vi "Slewing Test SAA.vi"(8 "error in (no error)":errorcluster, 10 "Model in":refnum<class "Model.lvclass">, 11 "Test Actuator State in":refnum<class "Test Actuator State.lvclass">) -> (0 "error out":errorcluster, 1 "Pass":bool, 2 "Model out":refnum<class "Model.lvclass">, 3 "Test Actuator State out":refnum<class "Test Actuator State.lvclass">)   [LabVIEW 2016, in "Test Actuator State.lvclass"]
uses:
  Test Actuator State.lvclass
  Model/Model/Model.lvclass
  <vilib>/Platform/TimedLoop/XDataNode/timing_clust.ctl
  <vilib>/Platform/TimedLoop/XDataNode/nitl_modes.ctl
  <vilib>/Platform/TimedLoop/XDataNode/wakeup.ctl
  Model/Model/Model.lvclass/Model.ctl
  Typedefs/ActuatorSetPoints.ctl
  <vilib>/Analysis/baseanly.llb/Mean (DBL).vi
  <vilib>/platform/TimedLoop/XDataNode/XDataNode.xnode
  Model/Waveforms/Waveform/Waveform.lvclass
  Typedefs/FAMT Typedefs.lvlib
  <vilib>/Analysis/NI_AALBase.lvlib
  <vilib>/Platform/TimedLoop/XDataNode/XDNodeRunTimeDep.lvlib
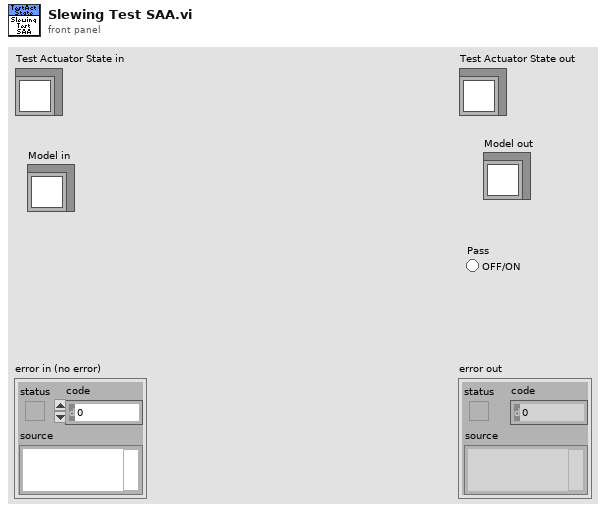
[diagram p1: front panel]
types:
  T1 = typedef "FAMT Typedefs.lvlib/SlewingTestSettings.ctl" = cluster{"Max Force Error (N)":dbl, "Max Moment (NM)":dbl, "Amplitude (N)":dbl, "Max Instance Force Error (N)":dbl, "Ramp Time (s)":dbl, "Hold Time (s)":dbl, "Settling Time (s)":dbl}
  T2 = typedef "XDNodeRunTimeDep.lvlib/timing_clust.ctl" = cluster{"Expected End [f-1]":u64, "Actual End [f-1]":u64, "Finished Late? [f-1]":bool, "Expected End [i-1]":u64, "Actual End [i-1]":u64, "Finished Late? [i-1]":bool, "Expected Start [i]":u64, "Actual Start [i]":u64, "Expected Start [f]":u64, "Actual Start [f]":u64, "Source Name":string, "Structure Name":string, "Period":i64, "Deadline":i64, "Offset":i64, "Start":i64, "Priority":i32, "Timeout":i32, "Mode":T3, "Wakeup Reason":T4, "Error":errorcluster, "Source Type":string, "Secondary Source Type":string, "Global End Time":u64, "Global Start Time":u64, "Frame Duration":u64, "Iteration Duration":u64, "Assigned CPU":i32, "I/O Scan Engine Mode":u32}
  T3 = typedef "XDNodeRunTimeDep.lvlib/nitl_modes.ctl" = enum32{"No Change", "Process missed periods, maintain original phase", "Discard missed periods, maintain original phase", "Process missed periods, ignore original phase", "Discard missed periods, ignore original phase"}
  T4 = typedef "XDNodeRunTimeDep.lvlib/wakeup.ctl" = enum32{"Normal", "Aborted", "Asynchronous wakeup", "Timing source error", "Timed loop error", "Timeout"}
  T5 = typedef "FAMT Typedefs.lvlib/ActuatorSetPoints.ctl" = cluster{"Axial Force":dbl, "Lateral Force":dbl, "FC1 Force":dbl, "FC2 Force":dbl}
  T6 = typedef "FAMT Typedefs.lvlib/ActuatorData.ctl" = cluster{"Timestamp":dbl, "Axial Force":dbl, "Lateral Force":dbl, "FC1 Force":dbl, "FC2 Force":dbl, "Lateral Push Pressure":dbl, "Lateral Pull Pressure":dbl, "Axial Push Pressure":dbl, "Axial Pull Pressure":dbl}
  T7 = typedef "FAMT Typedefs.lvlib/ToveyEngData.ctl" = cluster{"Timestamp":dbl, "Fx":dbl, "Fy":dbl, "Fz":dbl, "Mx":dbl, "My":dbl, "Mz":dbl}
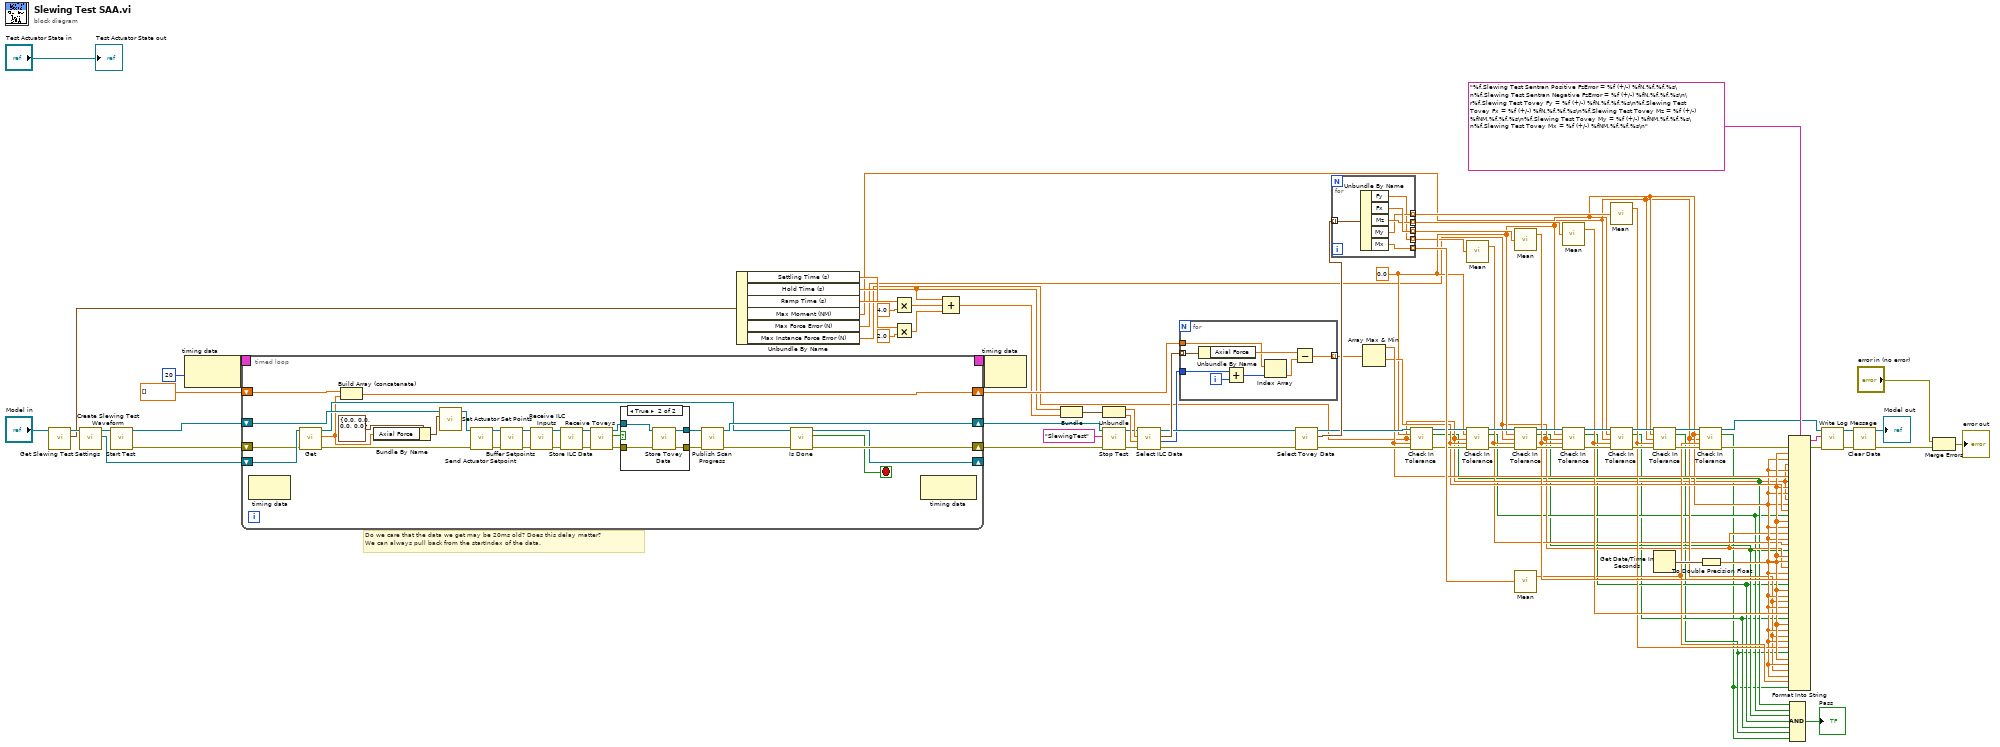
[diagram p0: block diagram]
diagram:
  w24 = 0.0
  # "Do we care that the data we get may be 20ms old? Does this delay matter?\nWe can always pull back from the startIndex of the data."
  n1 = call "Get Slewing Test Settings.vi"("Model in"="Model in") -> ("Slewing Test Settings"=w81:T1, "Model out"=w82:refnum<class "Model.lvclass">)  [unwired: 9 in]
  n2 = call "Create Slewing Test Waveform.vi"("Model in"=w82) -> ("Waveform"=w78:refnum<class "Waveform.lvclass">, "Model out"=w1:refnum<class "Model.lvclass">)  [unwired: 9 in]
  n3 = call "Start Test.vi"("Model in"=w1) -> ("error out"=w15:errorcluster, "Model out"=w16:refnum<class "Model.lvclass">)  [unwired: 9 in]
  n4 = node-c288(i64 20 ("Period")) -> (w73:T2)
  n5 = timed-loop {
    shift-right: [w113] -> w14
    shift-left: w16 -> [w105]
    shift-right: [w96] -> w13
    shift-left: w15 -> [w99]
    shift-right: [w94] -> _
    shift-left: w78 -> [w101]
    shift-right: [w91] -> w74
    shift-left: dbl[] [] -> [w93]
    timing: w73 -> [_]
    timing-out: [_] -> w72
    stop <- w95 stop-if-true
    n6 = node-c288() -> ()  [unwired: 1 in, 1 out]
    n7 = call-dynamic "Get.vi"("error in (no error)"=w99, "Waveform in"=w101) -> ("error out"=w98:errorcluster, "Value"=w92:dbl, "Waveform out"=w100:refnum<class "Waveform.lvclass">)  [unwired: 7 in]
    n8 = Build Array (concatenate)(w93, w92) -> (w91:dbl[])
    n9 = Bundle By Name(cluster=T5 {"Axial Force"=0.0, "Lateral Force"=0.0, "FC1 Force"=0.0, "FC2 Force"=0.0} ("Actuator Set Points"), "Axial Force"=w92) -> (w102:T5)
    n10 = call "Set Actuator Set Points.vi"("Actuator Set Points"=w102, "Model in"=w105) -> ("Model out"=w104:refnum<class "Model.lvclass">)  [unwired: 9 in]
    n11 = call "Send Actuator Setpoint.vi"("error in (no error)"=w98, "Model in"=w104) -> ("error out"=w88:errorcluster, "Model out"=w90:refnum<class "Model.lvclass">)  [unwired: 8 in]
    n12 = call "Buffer Setpoints.vi"("error in (no error)"=w88, "Model in"=w90) -> ("error out"=w87:errorcluster, "Model out"=w89:refnum<class "Model.lvclass">)  [unwired: 8 in]
    n13 = call "Receive ILC Inputs.vi"("error in (no error)"=w87, "Model in"=w89) -> ("error out"=w114:errorcluster, "Model out"=w115:refnum<class "Model.lvclass">)  [unwired: 8 in]
    n14 = call "Store ILC Data.vi"("error in (no error)"=w114, "Model in"=w115) -> ("error out"=w111:errorcluster, "Model out"=w112:refnum<class "Model.lvclass">)  [unwired: 8 in]
    n15 = call "Receive Toveys.vi"("error in (no error)"=w111, "Model in"=w112) -> ("error out"=w109:errorcluster, "Data Received"=w108:bool, "Model out"=w110:refnum<class "Model.lvclass">)  [unwired: 7 in]
    n16 = case shown="True" w108 {
      tunnel: w110 -> [w119 w123]
      tunnel: w109 -> [w118 w122]
      tunnel: [w118 w121] -> w106
      tunnel: [w119 w120] -> w107
      frame False {
      }
      frame True {
        n17 = call "Store Tovey Data.vi"("error in (no error)"=w122, "Model in"=w123) -> ("error out"=w121:errorcluster, "Model out"=w120:refnum<class "Model.lvclass">)  [unwired: 8 in]
      }
    }
    n18 = call "Publish Scan Progress.vi"("error in (no error)"=w106, "Model in"=w107) -> ("error out"=w97:errorcluster, "Model out"=w113:refnum<class "Model.lvclass">)  [unwired: 8 in]
    n19 = call-dynamic "Is Done.vi"("error in (no error)"=w97, "Waveform in"=w100) -> ("error out"=w96:errorcluster, "Is Done"=w95:bool, "Waveform out"=w94:refnum<class "Waveform.lvclass">)  [unwired: 7 in]
    n20 = node-c288() -> ()  [unwired: 1 in, 1 out]
  }
  n21 = Unbundle By Name(w81) -> ("Settling Time (s)"=w64:dbl, "Hold Time (s)"=w68:dbl, "Ramp Time (s)"=w70:dbl, "Max Moment (NM)"=w21:dbl, "Max Force Error (N)"=w17:dbl, "Max Instance Force Error (N)"=w20:dbl)
  n22 = Multiply(x=w70, y=4.0) -> (x*y=w66:dbl)
  n23 = Multiply(x=w68, y=2.0) -> (x*y=w65:dbl)
  n24 = Compound Arithmetic op=ADD(w64, w66, w65) -> (w63:dbl)
  n25 = node-c288(w72) -> ()  [unwired: 1 out]
  n26 = Bundle("Settling Time (s)"=w64, w63) -> (w62:cluster{"Settling Time (s)":dbl, dbl})  [unwired: 1 in]
  n27 = Unbundle(w62) -> ("Settling Time (s)"=w23:dbl, w22:dbl)
  n28 = call "Stop Test.vi"("error in (no error)"=w13, "Test"="SlewingTest", "Model in"=w14) -> ("error out"=w12:errorcluster, "Model out"=w11:refnum<class "Model.lvclass">)  [unwired: 7 in]
  n29 = call "Select ILC Data.vi"("error in (no error)"=w12, "End Time"=w22, "Start Time"=w23, "Model in"=w11) -> ("error out"=w59:errorcluster, "StartIndex"=w47:i32, "Data"=w61:T6[], "Model out"=w60:refnum<class "Model.lvclass">)  [unwired: 4 in]
  n30 = for {
    tunnel: w61 -> [w131] mode=indexing
    tunnel: [w129] -> w46 mode=indexing
    tunnel: w74 -> [w125]
    tunnel: w47 -> [w128]
    i -> [w127]
    n31 = Unbundle By Name(w131) -> ("Axial Force"=w130:dbl)
    n32 = Add(x=w128, y=w127) -> (x+y=w126:i32)
    n33 = Index Array(array=w125, index=w126) -> (element=w124:dbl)
    n34 = Subtract(x=w130, y=w124) -> (x-y=w129:dbl)
  }
  n35 = call "Select Tovey Data.vi"("error in (no error)"=w59, "Model in"=w60) -> ("error out"=w54:errorcluster, "Data"=w58:T7[], "Model out"=w55:refnum<class "Model.lvclass">)  [unwired: 6 in, 1 out]
  n36 = for {
    tunnel: [w137] -> w51 mode=indexing
    tunnel: [w136] -> w50 mode=indexing
    tunnel: [w135] -> w49 mode=indexing
    tunnel: [w134] -> w48 mode=indexing
    tunnel: w58 -> [w133] mode=indexing
    tunnel: [w132] -> w19 mode=indexing
    n37 = Unbundle By Name(w133) -> ("Fy"=w132:dbl, "Fx"=w137:dbl, "Mz"=w136:dbl, "My"=w135:dbl, "Mx"=w134:dbl)
  }
  n38 = Array Max & Min(array=w46) -> (max value=w31:dbl, min value=w30:dbl)  [unwired: 2 out]
  n39 = call "Check In Tolerance.vi"("Model in"=w55, "Expected"=w24, "Tolerance"=w20, "Actual"=w31, "error in (no error)"=w54) -> ("Model out"=w42:refnum<class "Model.lvclass">, "Pass"=w9:bool, "error out"=w45:errorcluster)  [unwired: 8 in]
  n40 = call-poly <vilib>:"Mean.vi"("X"=w19) -> ("mean"=w18:dbl)  [unwired: 1 out]
  n41 = call "Check In Tolerance.vi"("Model in"=w42, "Expected"=w24, "Tolerance"=w20, "Actual"=w30, "error in (no error)"=w45) -> ("Model out"=w41:refnum<class "Model.lvclass">, "Pass"=w8:bool, "error out"=w44:errorcluster)  [unwired: 8 in]
  n42 = call-poly <vilib>:"Mean.vi"("X"=w51) -> ("mean"=w29:dbl)  [unwired: 1 out]
  n43 = call "Check In Tolerance.vi"("Model in"=w41, "Expected"=w24, "Tolerance"=w17, "Actual"=w18, "error in (no error)"=w44) -> ("Model out"=w40:refnum<class "Model.lvclass">, "Pass"=w7:bool, "error out"=w43:errorcluster)  [unwired: 8 in]
  n44 = call-poly <vilib>:"Mean.vi"("X"=w48) -> ("mean"=w26:dbl)  [unwired: 1 out]
  n45 = call-poly <vilib>:"Mean.vi"("X"=w50) -> ("mean"=w28:dbl)  [unwired: 1 out]
  n46 = call "Check In Tolerance.vi"("Model in"=w40, "Expected"=w24, "Tolerance"=w17, "Actual"=w29, "error in (no error)"=w43) -> ("Model out"=w33:refnum<class "Model.lvclass">, "Pass"=w6:bool, "error out"=w39:errorcluster)  [unwired: 8 in]
  n47 = call-poly <vilib>:"Mean.vi"("X"=w49) -> ("mean"=w25:dbl)  [unwired: 1 out]
  n48 = call "Check In Tolerance.vi"("Model in"=w33, "Expected"=w24, "Tolerance"=w21, "Actual"=w28, "error in (no error)"=w39) -> ("Model out"=w34:refnum<class "Model.lvclass">, "Pass"=w5:bool, "error out"=w38:errorcluster)  [unwired: 8 in]
  n49 = call "Check In Tolerance.vi"("Model in"=w34, "Expected"=w24, "Tolerance"=w21, "Actual"=w25, "error in (no error)"=w38) -> ("Model out"=w35:refnum<class "Model.lvclass">, "Pass"=w4:bool, "error out"=w37:errorcluster)  [unwired: 8 in]
  n50 = Get Date/Time In Seconds() -> (seconds since 1Jan1904=w56:timestamp)
  n51 = call "Check In Tolerance.vi"("Model in"=w35, "Expected"=w24, "Tolerance"=w21, "Actual"=w26, "error in (no error)"=w37) -> ("Model out"=w32:refnum<class "Model.lvclass">, "Pass"=w3:bool, "error out"=w36:errorcluster)  [unwired: 8 in]
  n52 = To Double Precision Float(number=w56) -> (double precision float=w27:dbl)
  n53 = Format Into String(format string="%f,Slewing Test Sentran Positive FzError = %f (+/-) %fN,%f,%f,%s\n%f,Slewing Test Sentran Negative FzError = %f (+/-) %fN,%f,%f,%s\n\r%f,Slewing Test Tovey Fy = %f (+/-) %fN,%f,%f,%s\n%f,Slewing Test Tovey Fx = %f (+/-) %fN,%f,%f,%s\n%f,Slewing Test Tovey Mz = %f (+/-) %fNM,%f,%f,%s\n%f,Slewing Test Tovey My = %f (+/-) %fNM,%f,%f,%s\n%f,Slewing Test Tovey Mx = %f (+/-) %fNM,%f,%f,%s\n", error in=w36, w27, w24, w20, w24, w31, w9, w27, w24, w20, w24, w30, w8, w27, w24, w17, w24, w18, w7, w27, w24, w17, w24, w29, w6, w27, w24, w21, w24, w28, w5, w27, w24, w21, w24, w25, w4, w27, w24, w21, w24, w26, w3) -> (resulting string=w52:string, error out=w53:errorcluster)  [unwired: 1 in]
  n54 = Compound Arithmetic op=AND(w9, w8, w7, w6, w5, w4, w3) -> (→"Pass":bool)
  n55 = call "Write Log Message.vi"("error in (no error)"=w53, "Message"=w52, "Model in"=w32) -> ("error out"=w77:errorcluster, "Model out"=w76:refnum<class "Model.lvclass">)  [unwired: 7 in]
  n56 = call "Clear Data.vi"("error in (no error)"=w77, "Model in"=w76) -> ("error out"=w80:errorcluster, "Model out"=→"Model out":refnum<class "Model.lvclass">)  [unwired: 8 in]
  n57 = Merge Errors("error in (no error)", w80) -> (→"error out":errorcluster)
  "Test Actuator State out" <- "Test Actuator State in"
